vi "Send Event Msg.vi"(8 "error in":errorcluster, 10 "event":T1, 11 "Qbus in":refnum<class "Qbus.lvclass">) -> (0 "error out":errorcluster, 3 "Qbus out":refnum<class "Qbus.lvclass">)   [LabVIEW 2021, in "EventLoggerProcess.lvlib"]
uses:
  EventLoggerProcess.lvlib
  <vilib>/addons/Qbus/Qbus.lvclass
  controls/event.ctl
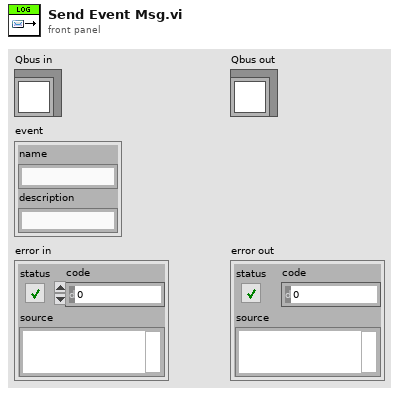
[diagram p1: front panel]
types:
  T1 = typedef "EventLoggerProcess.lvlib/event.ctl" = cluster{"name":string, "description":string}
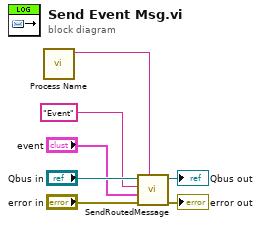
[diagram p0: block diagram]
diagram:
  n1 = call "Process Name.vi"() -> ("process name"=w3:string)  [unwired: 11 in]
  n2 = call <vilib>:"SendRoutedMessage.vi"("listener process"=w3, "error in (no error)"="error in", "message value"="event", "message name"="Event", "Qbus in"="Qbus in") -> ("error in (no error)"=→"error out":errorcluster, "Qbus out"=→"Qbus out":refnum<class "Qbus.lvclass">)  [unwired: 5 in]
